vi "Write Metadata to SnP File.vi"(0 "SnP File Path in":path, 5 "Key":string, 7 "Value":string, 11 "error in (no error)":errorcluster) -> (4 "SnP File Path out":path, 15 "error out":errorcluster)   [LabVIEW 2023, in "RFFixtureCharact.RFPM.lvlib" / "Charact Result Accessor.lvclass"]
uses:
  Charact Result Accessor.lvclass
  Global IDs.vi
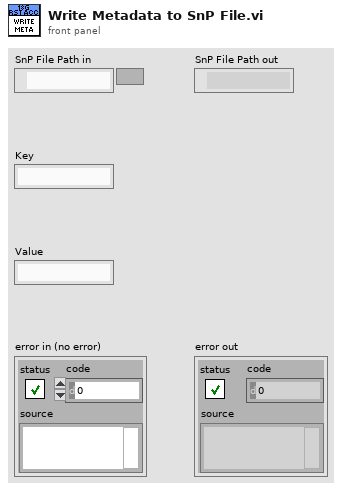
[diagram p1: front panel]
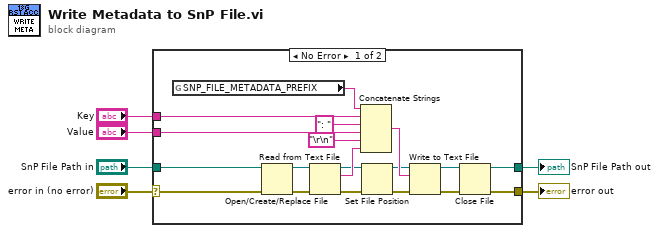
[diagram p0: block diagram]
diagram:
  n1 = case shown="No Error" "error in (no error)" {
    selector: "error in (no error)" -> [w7 w27]
    tunnel: [w25 w27] -> w5
    tunnel: "SnP File Path in" -> [w16 w26]
    tunnel: [w19 w26] -> w3
    tunnel: "Key" -> [w10 _]
    tunnel: "Value" -> [w8 _]
    frame No Error {
      n2 = global read "Global IDs.vi" "SNP_FILE_METADATA_PREFIX"() -> (w18:string)
      n3 = Open/Create/Replace File(file path (use dialog)=w16, error in=w7) -> (refnum out=w15:refnum<file>, error out=w17:errorcluster)  [unwired: 4 in, 1 out]
      n4 = Read from Text File(file (use dialog)=w15, error in=w17) -> (refnum out=w12:refnum<file>, text=w21:string, error out=w14:errorcluster)  [unwired: 2 in, 1 out]
      n5 = Concatenate Strings(w18, w10, ": " ("string"), w8, "\r\n", w21) -> (w20:string)
      n6 = Set File Position(refnum=w12, error in=w14) -> (refnum out=w11:refnum<file>, error out=w13:errorcluster)  [unwired: 2 in]
      n7 = Write to Text File(file (use dialog)=w11, text=w20, error in=w13) -> (refnum out=w23:refnum<file>, error out=w24:errorcluster)  [unwired: 1 in, 1 out]
      n8 = Close File(refnum=w23, error in=w24) -> (path=w19:path, error out=w25:errorcluster)
    }
    frame Error {
    }
  }
  "error out" <- w5
  "SnP File Path out" <- w3
